vi "Write Lambda.vi"(8 "error in (no error)":errorcluster, 10 "Lambda":dbl, 11 "Scheduler in":refnum<class "Scheduler.lvclass">) -> (0 "error out":errorcluster, 3 "Scheduler out":refnum<class "Scheduler.lvclass">)   [LabVIEW 2013, in "Scheduler.lvclass"]
uses:
  Scheduler.lvclass
  Scheduler.lvclass/Scheduler.ctl
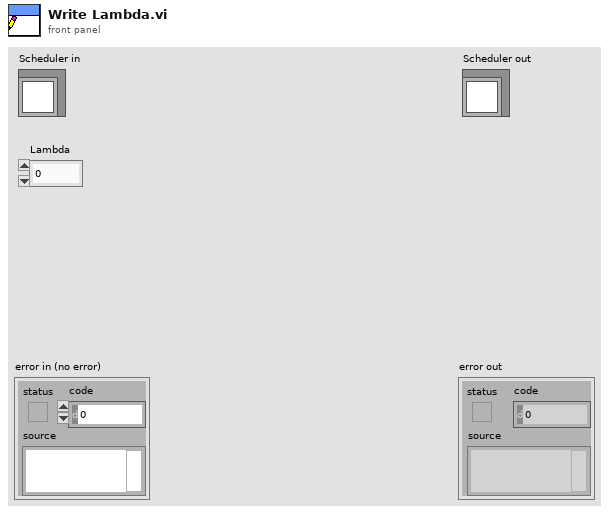
[diagram p1: front panel]
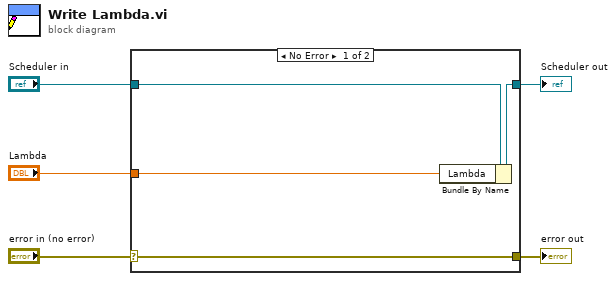
[diagram p0: block diagram]
diagram:
  n1 = case shown="No Error" "error in (no error)" {
    selector: "error in (no error)" -> [w9 w10]
    tunnel: [w9 w10] -> w4
    tunnel: [w7 w11] -> w2
    tunnel: "Scheduler in" -> [w8 w11]
    tunnel: "Lambda" -> [w6 _]
    frame No Error {
      n2 = Bundle By Name(cluster=w8, "Lambda"=w6) -> (w7:refnum<class "Scheduler.lvclass">)
    }
    frame Error {
    }
  }
  "error out" <- w4
  "Scheduler out" <- w2
